vi "Find Number of Knobs.vi"(0 "Test Results In":T1, 11 "error in (no error)":errorcluster) -> (4 "Test Results Out":T1, 6 "Pass/Fail?":bool, 8 "Report Text":string, 10 "Number of Knobs":i32, 15 "error out":errorcluster)   [LabVIEW 2016]
doc: "This VI searches the config file for the hardware type defined by model number in the Model Config file."
uses:
  controls/Test Results.ctl
  <vilib>/Utility/config.llb/Read Key (String).vi
  <vilib>/Utility/error.llb/Error Cluster From Error Code.vi
  <vilib>/ErrorRing/Error Ring.xnode
  <vilib>/Utility/config.llb/NI_LVConfig.lvlib
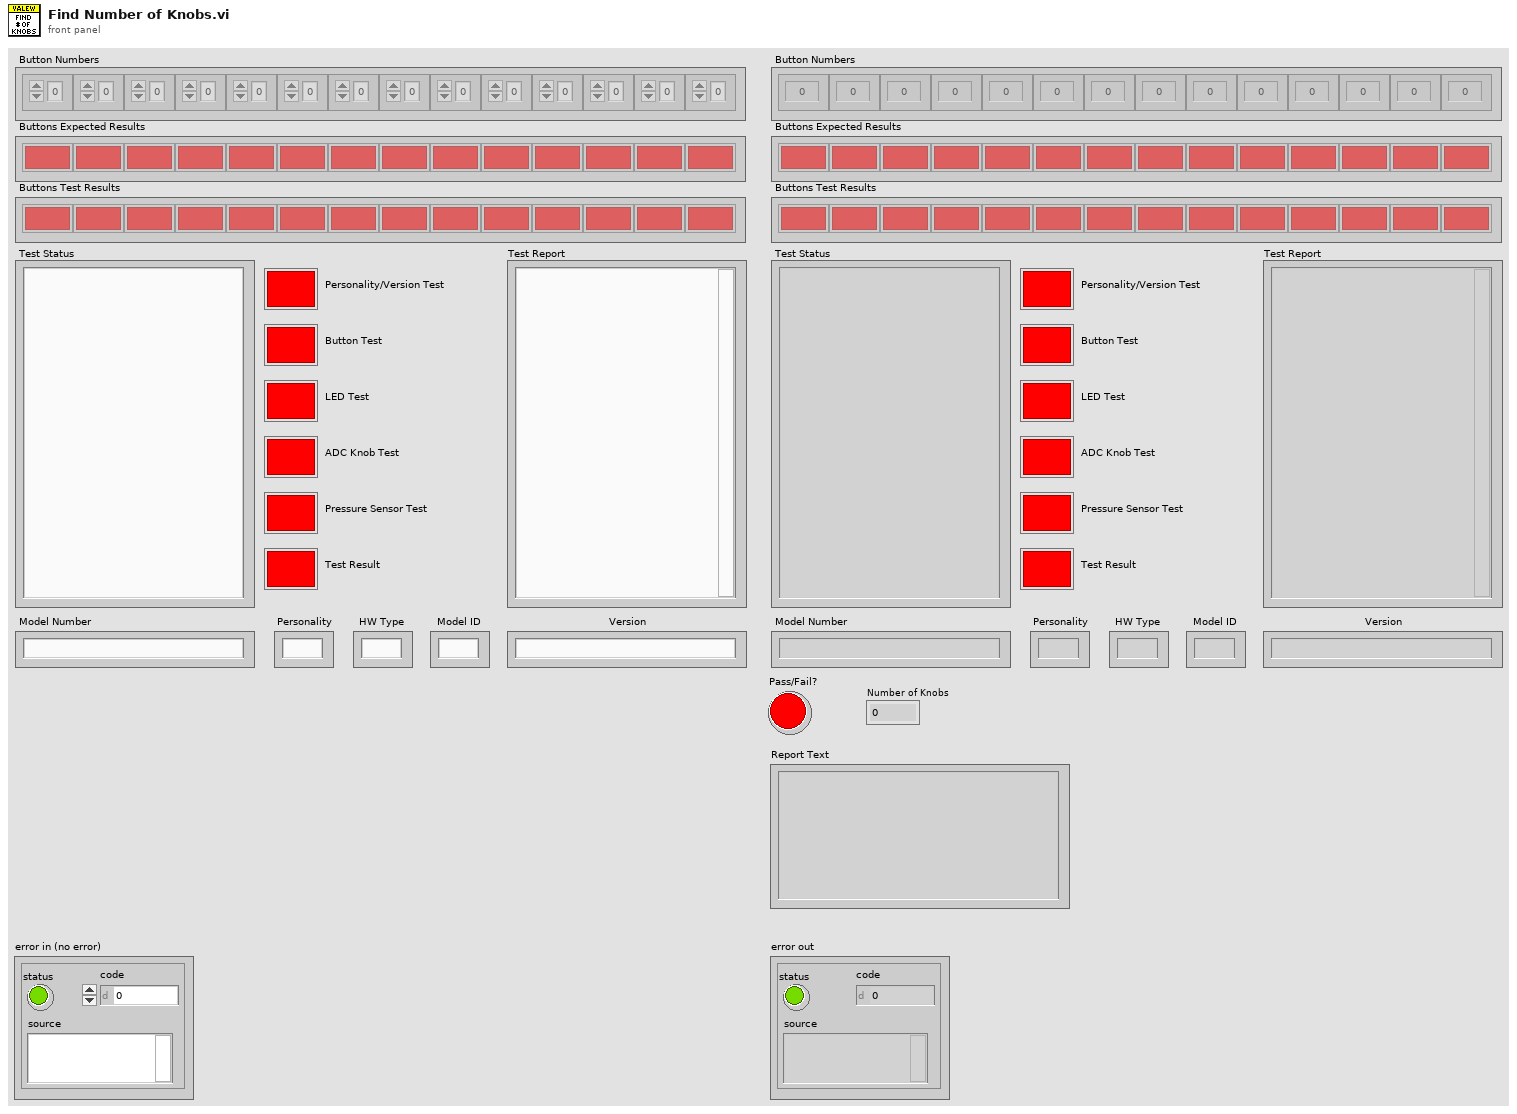
[diagram p1: front panel]
types:
  T1 = typedef "Test Results.ctl" = cluster{"Test Status":string, "Personality/Version Test ":bool, "Test Report":string, "Model Number":string, "Button Numbers":i32[], "Buttons Test Results":bool[], "Buttons Expected Results":bool[], "Model ID":string, "Personality":string, "HW Type":string, "Version":string, "Button Test":bool, "LED Test":bool, "ADC Knob Test":bool, "Pressure Sensor Test":bool, "Test Result":bool}
  T2 = typedef "NI_LVConfig.lvlib/Config Data RefNum.ctl" = refnum<k1>
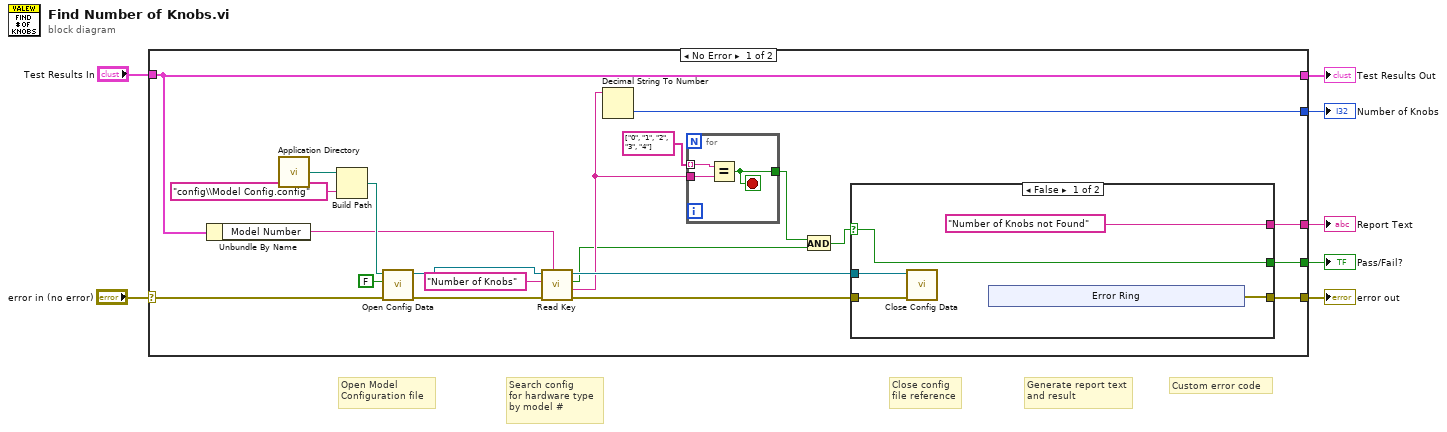
[diagram p0: block diagram]
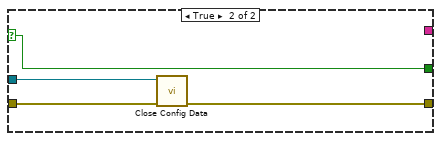
[diagram p2: hidden frame]
diagram:
  # "Custom error code"
  # "Generate report text\nand result"
  # "Close config\nfile reference"
  # "Search config \nfor hardware type\nby model #"
  # "Open Model \nConfiguration file"
  n1 = case shown="No Error" "error in (no error)" {
    selector: "error in (no error)" -> [w18 w46]
    tunnel: [w27 w46] -> w7
    tunnel: [w17 _] -> w5
    tunnel: [w16 _] -> w4
    tunnel: "Test Results In" -> [w14 _]
    tunnel: [w14 _] -> w2
    tunnel: [w13 _] -> w1
    frame No Error {
      n2 = Unbundle By Name(w14) -> ("Model Number"=w15:string)
      n3 = call <vilib>:"Application Directory.vi"() -> ("Application Directory"=w23:path)
      n4 = Build Path(base path=w23, name or relative path="config\\Model Config.config") -> (appended path=w22:path)
      n5 = call <vilib>:"Open Config Data.vi"("error in (no error)"=w18, "create file if necessary (T)"=FALSE, "configuration file path"=w22) -> ("error out"=w21:errorcluster, "refnum"=w19:T2)  [unwired: 6 in, 1 out]
      n6 = call-poly <vilib>:"Read Key.vi"("section"=w15, "error in (no error)"=w21, "key"="Number of Knobs", "refnum"=w19) -> ("error out"=w28:errorcluster, "value"=w11:string, "found?"=w8:bool, "refnum out"=w26:T2)  [unwired: 4 in]
      n7 = Decimal String To Number(string=w11) -> (number=w13:i32)  [unwired: 2 in, 1 out]
      n8 = for {
        tunnel: w11 -> [w31]
        tunnel: string[] ["0", "1", "2", "3", "4"] -> [w30] mode=indexing
        tunnel: [w29] -> w10
        stop <- w29 stop-if-true
        n9 = Equal?(x=w30, y=w31) -> (x = y?=w29:bool)
      }
      n10 = And(x=w10, y=w8) -> (x .and. y?=w9:bool)
      n11 = case shown="False" w9 {
        selector: w9 -> [w35 w42]
        tunnel: w28 -> [w33 w45]
        tunnel: [w36 w44] -> w27
        tunnel: w26 -> [w32 w43]
        tunnel: [w35 w42] -> w17
        tunnel: ["Number of Knobs not Found" _] -> w16
        frame False {
          n12 = call <vilib>:"Close Config Data.vi"("error in (no error)"=w33, "refnum"=w32) -> ()  [unwired: 8 in, 2 out]
          n13 = xnode "Error Ring"() -> ("error out"=w36:errorcluster)
        }
        frame True {
          n14 = call <vilib>:"Close Config Data.vi"("error in (no error)"=w45, "refnum"=w43) -> ("error out"=w44:errorcluster)  [unwired: 8 in, 1 out]
        }
      }
    }
    frame Error {
    }
  }
  "error out" <- w7
  "Report Text" <- w4
  "Pass/Fail?" <- w5
  "Test Results Out" <- w2
  "Number of Knobs" <- w1
